vi "Untitled 1.vi"   [LabVIEW 2014]
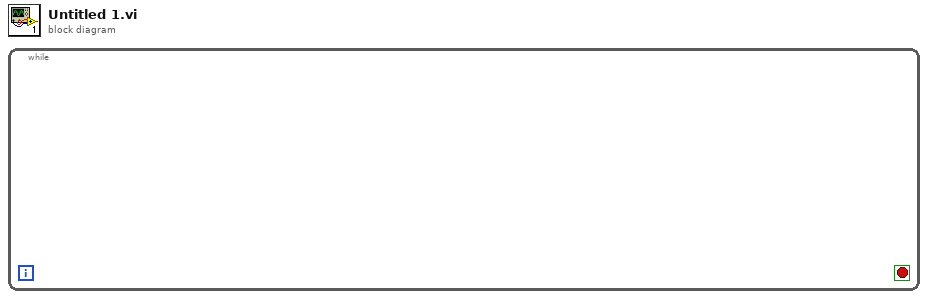
[diagram p0: block diagram]
diagram:
  n1 = while {
    stop <- _ stop-if-true
  }
